vi "三维坐标系变换.vi"() -> ()   [LabVIEW 2018]
uses:
  <vilib>/Analysis/coordinate.llb/3D Coordinate Conversion (Array).vi
  <vilib>/Analysis/NI_AALPro.lvlib
panel:
  out "Axis 2 Out":dbl[](array[numeric]) caption="坐标轴2输出"
  out "Axis 3 Out":dbl[](array[numeric]) caption="坐标轴3输出"
  out "Axis 1 Out":dbl[](array[numeric]) caption="坐标轴1输出"
  in  "Axis 3":dbl[](array[numeric]) caption="坐标轴3"
  in  "Axis 2":dbl[](array[numeric]) caption="坐标轴2"
  in  "Axis 1":dbl[](array[numeric]) caption="坐标轴1"
  in  "conversion type":u16(ring) caption="转换类型" items=["直角坐标至球坐标转换", "球坐标至直角坐标转换", "直角坐标至柱坐标转换", "柱坐标至直角坐标转换", "球坐标至柱坐标转换", "柱坐标至球坐标转换"]
  in  "停止":bool
  out "说明":string="三维坐标系变换是在直角坐标、柱坐标、球坐标之间变换"
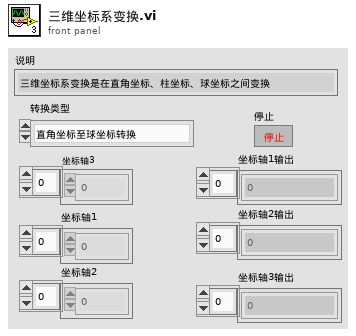
[diagram p1: front panel]
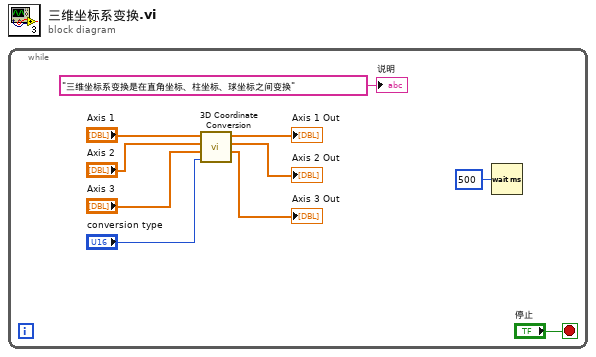
[diagram p0: block diagram]
diagram:
  n1 = while {
    stop <- "停止" stop-if-true
    n2 = call-poly <vilib>:"3D Coordinate Conversion.vi"("conversion type"="conversion type", "Axis 3"="Axis 3", "Axis 2"="Axis 2", "Axis 1"="Axis 1") -> ("Axis 3 Out"=→"Axis 3 Out":dbl[], "Axis 2 Out"=→"Axis 2 Out":dbl[], "Axis 1 Out"=→"Axis 1 Out":dbl[])  [unwired: 4 in, 1 out]
    n3 = Wait (ms)(milliseconds to wait=u32 500 ("等待时间（毫秒）")) -> ()  [unwired: 1 out]
    "说明" <- "三维坐标系变换是在直角坐标、柱坐标、球坐标之间变换"
  }
